vi "Controller Response Matrix Measurement Loop.vi"(7 "Sync Objects":T1, 8 "error in (no error)":errorcluster, 11 "FOFB Configuration":T5={"FOFB Parameters"={"Network"={"FOFB Controller IP"="", "LNLS Control Network IP"="", "LNLS Control Network Power Supplies TCP Port"=0, "LNLS Control Network FOFB Configuration TCP Port"=0, "Data Server TCP Port"=0, "Monitoring Data TCP Port"=0, "Configuration GUI TCP Port"=0, "TCP Listening Timeout"=0}, "Fast Acquisition"={"Acquisition Period"=0, "Data Buffer Size"=0}, "Response Matrix Measurement"={"Step Amplitude"=0.0, "Time Between Steps"=0, "Step Duration"=0, "Number of Averages"=0}, "Correction Algorithm"={"Correction Period"=0, "Reference Orbit Path"=path "", "Response Matrix Path"=path "", "Correction Matrix Path"=path "", "Horizontal Correction Factor"=0.0, "Vertical Correction Factor"=0.0, "Beam Current FOFB Threshold"=0.0, "Decouple H-V"=FALSE}, "Acquisition Network"=[], "Actuation Network"=[]}, "Number of Acquisition Chassis"=0, "Number of Actuation Chassis"=0, "Number of BPM Readings"=0, "BPM Reading Names"=[], "Selected BPM Readings"=[0, 1, 2, 3, 4, 5, 6, 7, 8, 9, 10, 11, 12, 13, 14, 15, 16, 17, 18, 19, 20, 21, 22, 23, 24, 25, 26, 27, 28, 29, 30, 31, 32, 33, 34, 35, 36, 37, 38, 39, 40, 41, 42, 43, 44, 45, 46, 47, 48, 49], "Number of Correctors"=0, "Corrector Names"=[], "Selected Correctors"=[0, 1, 2, 3, 4, 5, 6, 7, 8, 9, 10, 11, 12, 13, 14, 15, 16, 17, 18, 19, 20, 21, 22, 23, 24, 25, 26, 27, 28, 29, 30, 31, 32, 33, 34, 35, 36, 37, 38, 39, 40, 41, 42, 43, 44, 45, 46, 47, 48, 49], "Reference Orbit"=[], "Response Matrix"=[], "Correction Matrix"=[], "Acquisition Chassis Names"=[], "Actuation Chassis Names"=[], "Acquisition Variables"=[], "Actuation Variables"=[], "PS Matrix Mapping"=[], "Inverse PS Matrix Mapping"=[], "Response Matrix Beam Energy (MeV)"=0.0, "PID Parameters"=[], "BPM Planes"=[], "Corrector Planes"=[], "RMM Step Factor"=[]}) -> (0 "error out":errorcluster)   [LabVIEW 2011, in "Controller VIs.lvlib"]
uses:
  Controller VIs.lvlib
  Types Definitions/Type FOFB Configuration.ctl
  Types Definitions/Type FOFB Parameters.ctl
  Types Definitions/Type Network Configuration.ctl
  Types Definitions/Type FA Configuration.ctl
  Types Definitions/Type Response Matrix Measurement Configuration.ctl
  Types Definitions/Type Correction Algorithm Configuration.ctl
  Types Definitions/Type Acquisition Network Configuration.ctl
  Types Definitions/Type Actuation Network Configuration.ctl
  Types Definitions/Type PID Parameters.ctl
  Types Definitions/Type Synchronization Objects.ctl
  Types Definitions/Type Blocking Synchronization Objects.ctl
  Types Definitions/Type FA Request Parameters.ctl
  Types Definitions/Type BPM and PS select cluster.ctl
  Types Definitions/Type FA File Parameters.ctl
  Types Definitions/Type Monitoring Data.ctl
  Types Definitions/Type Diagnostics Data.ctl
  Types Definitions/Type CPU Loads Array.ctl
  Types Definitions/Type CPU Loads.ctl
  Types Definitions/Type Non-blocking Synchronization Objects.ctl
  Types Definitions/Type FOFB Variables.ctl
  Types Definitions/Type Actuation State.ctl
  <vilib>/Platform/TimedLoop/XDataNode/timing_clust.ctl
  <vilib>/Platform/TimedLoop/XDataNode/nitl_modes.ctl
  <vilib>/Platform/TimedLoop/XDataNode/wakeup.ctl
  Controller Global Variables/Monitoring Data.vi
  Controller Global Variables/LNLS Control FOFB Configuration Out.vi
  <vilib>/Platform/TimedLoop/XDataNode/XDataNode.xnode
  File VIs.lvlib
  Controller Global Variables.lvlib
  Type Definitions.lvlib
  <vilib>/Platform/TimedLoop/XDataNode/XDNodeRunTimeDep.lvlib
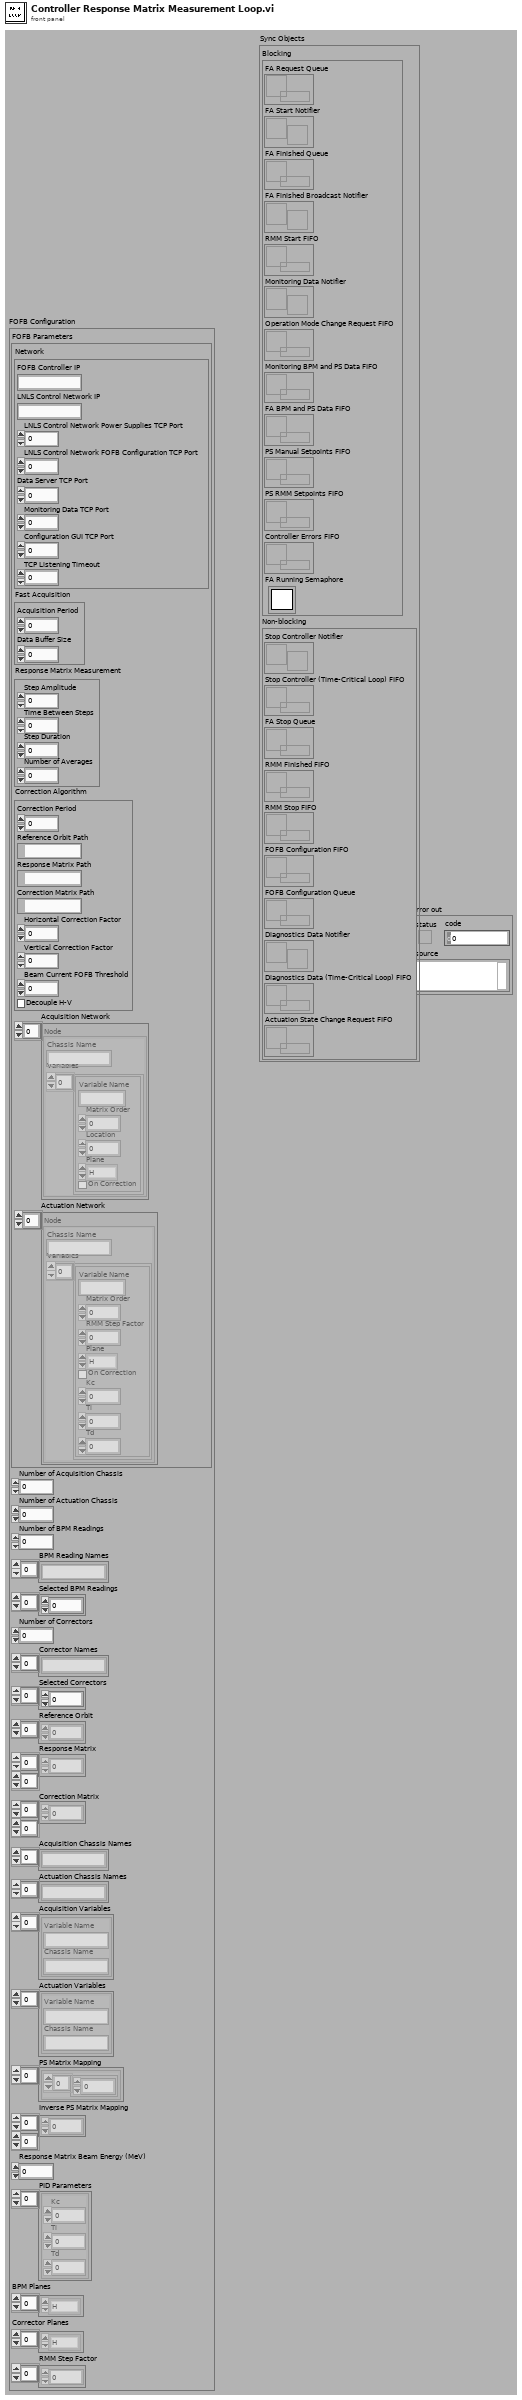
[diagram p1: front panel]
types:
  T1 = typedef "Type Definitions.lvlib/Type Synchronization Objects.ctl" = cluster{"Blocking":T2, "Non-blocking":T4}
  T2 = typedef "Type Definitions.lvlib/Type Blocking Synchronization Objects.ctl" = cluster{"FA Request Queue":refnum<queue>, "FA Start Notifier":refnum<notifier>, "FA Finished Queue":refnum<queue>, "FA Finished Broadcast Notifier":refnum<notifier>, "RMM Start FIFO":refnum<k33>, "Monitoring Data Notifier":refnum<notifier>, "Operation Mode Change Request FIFO":refnum<k33>, "Monitoring BPM and PS Data FIFO":refnum<k33>, "FA BPM and PS Data FIFO":refnum<k33>, "PS Manual Setpoints FIFO":refnum<k33>, "PS RMM Setpoints FIFO":refnum<k33>, "Controller Errors FIFO":refnum<k33>, "FA Running Semaphore":T3}
  T3 = typedef "Semaphore RefNum" = refnum<k1>
  T4 = typedef "Type Definitions.lvlib/Type Non-blocking Synchronization Objects.ctl" = cluster{"Stop Controller Notifier":refnum<notifier>, "Stop Controller (Time-Critical Loop) FIFO":refnum<k33>, "FA Stop Queue":refnum<queue>, "RMM Finished FIFO":refnum<k33>, "RMM Stop FIFO":refnum<k33>, "FOFB Configuration FIFO":refnum<k33>, "FOFB Configuration Queue":refnum<queue>, "Diagnostics Data Notifier":refnum<notifier>, "Diagnostics Data (Time-Critical Loop) FIFO":refnum<k33>, "Actuation State Change Request FIFO":refnum<k33>}
  T5 = typedef "Type Definitions.lvlib/Type FOFB Configuration.ctl" = cluster{"FOFB Parameters":T6, "Number of Acquisition Chassis":i32, "Number of Actuation Chassis":i32, "Number of BPM Readings":i32, "BPM Reading Names":string[], "Selected BPM Readings":u32[], "Number of Correctors":i32, "Corrector Names":string[], "Selected Correctors":u32[], "Reference Orbit":dbl[], "Response Matrix":dbl[][], "Correction Matrix":dbl[][], "Acquisition Chassis Names":string[], "Actuation Chassis Names":string[], "Acquisition Variables":cluster{"Variable Name":string, "Chassis Name":string}[], "Actuation Variables":cluster{"Variable Name":string, "Chassis Name":string}[], "PS Matrix Mapping":cluster{u32[]}[], "Inverse PS Matrix Mapping":u32[][], "Response Matrix Beam Energy (MeV)":dbl, "PID Parameters":T13[], "BPM Planes":enum8{"H", "V"}[], "Corrector Planes":enum8{"H", "V"}[], "RMM Step Factor":dbl[]}
  T6 = typedef "Type Definitions.lvlib/Type FOFB Parameters.ctl" = cluster{"Network":T7, "Fast Acquisition":T8, "Response Matrix Measurement":T9, "Correction Algorithm":T10, "Acquisition Network":T11, "Actuation Network":T12}
  T7 = typedef "Type Definitions.lvlib/Type Network Configuration.ctl" = cluster{"FOFB Controller IP":string, "LNLS Control Network IP":string, "LNLS Control Network Power Supplies TCP Port":u16, "LNLS Control Network FOFB Configuration TCP Port":u16, "Data Server TCP Port":u16, "Monitoring Data TCP Port":u16, "Configuration GUI TCP Port":u16, "TCP Listening Timeout":i32}
  T8 = typedef "Type Definitions.lvlib/Type FA Configuration.ctl" = cluster{"Acquisition Period":u32, "Data Buffer Size":u32}
  T9 = typedef "Type Definitions.lvlib/Type Response Matrix Measurement Configuration.ctl" = cluster{"Step Amplitude":dbl, "Time Between Steps":u32, "Step Duration":u32, "Number of Averages":u32}
  T10 = typedef "Type Definitions.lvlib/Type Correction Algorithm Configuration.ctl" = cluster{"Correction Period":u32, "Reference Orbit Path":path, "Response Matrix Path":path, "Correction Matrix Path":path, "Horizontal Correction Factor":dbl, "Vertical Correction Factor":dbl, "Beam Current FOFB Threshold":dbl, "Decouple H-V":bool}
  T11 = typedef "Type Definitions.lvlib/Type Acquisition Network Configuration.ctl" = cluster{"Chassis Name":string, "Variables":cluster{"Variable Name":string, "Matrix Order":u32, "Location":dbl, "Plane":enum8{"H", "V"}, "On Correction":bool}[]}[]
  T12 = typedef "Type Definitions.lvlib/Type Actuation Network Configuration.ctl" = cluster{"Chassis Name":string, "Variables":cluster{"Variable Name":string, "Matrix Order":u32, "RMM Step Factor":dbl, "Plane":enum8{"H", "V"}, "On Correction":bool, "Kc":dbl, "Ti":dbl, "Td":dbl}[]}[]
  T13 = typedef "Type Definitions.lvlib/Type PID Parameters.ctl" = cluster{"Kc":fxp<+/-,16,8>, "Ti":fxp<+/-,16,8>, "Td":fxp<+/-,16,8>}
  T14 = typedef "XDNodeRunTimeDep.lvlib/timing_clust.ctl" = cluster{"Expected End [f-1]":u64, "Actual End [f-1]":u64, "Finished Late? [f-1]":bool, "Expected End [i-1]":u64, "Actual End [i-1]":u64, "Finished Late? [i-1]":bool, "Expected Start [i]":u64, "Actual Start [i]":u64, "Expected Start [f]":u64, "Actual Start [f]":u64, "Source Name":string, "Structure Name":string, "Period":i64, "Deadline":i64, "Offset":i64, "Start":i64, "Priority":i32, "Timeout":i32, "Mode":T15, "Wakeup Reason":T16, "Error":errorcluster, "Source Type":string, "Secondary Source Type":string, "Global End Time":u64, "Global Start Time":u64, "Frame Duration":u64, "Iteration Duration":u64, "Assigned CPU":i32, "I/O Scan Engine Mode":u32}
  T15 = typedef "XDNodeRunTimeDep.lvlib/nitl_modes.ctl" = enum32{"No Change", "Process missed periods, maintain original phase", "Discard missed periods, maintain original phase", "Process missed periods, ignore original phase", "Discard missed periods, ignore original phase"}
  T16 = typedef "XDNodeRunTimeDep.lvlib/wakeup.ctl" = enum32{"Normal", "Aborted", "Asynchronous wakeup", "Timing source error", "Timed loop error", "Timeout"}
  T17 = typedef "Type Definitions.lvlib/Type BPM and PS select cluster.ctl" = cluster{"BPM index array":u32[], "PS index array ":u32[]}
  T18 = typedef "Type Definitions.lvlib/Type FA Request Parameters.ctl" = cluster{"Number of Samples":u32, "BPM and PS Selection":T17, "Filename":string}
  T19 = typedef "Type Definitions.lvlib/Type Monitoring Data.ctl" = cluster{"Timestamp":timestamp, "BPM Readings":dbl[], "PS Readings":dbl[], "PS FOFB Setpoints":dbl[], "PS Status per Rack":u8[], "PS ON-OFF per Rack":u8[], "Operation Mode":enum16{"Idle Mode", "Error Mode", "Manual Mode", "FOFB Mode", "RMM Mode"}, "Diagnostics Data":T20, "Controller Status Table":i32[]}
  T20 = typedef "Type Definitions.lvlib/Type Diagnostics Data.ctl" = cluster{"Time-Critical Loop Missed Iterations":u32, "Time-Critical Loop Execution Time (usec)":u32, "FA Buffer Usage":u32, "Available Memory (bytes)":u32, "CPU Loads Array":T21}
  T21 = typedef "Type Definitions.lvlib/Type CPU Loads Array.ctl" = T22[]
  T22 = typedef "Type Definitions.lvlib/Type CPU Loads.ctl" = cluster{"Total (%)":dbl, "Time Critical (%)":dbl, "Timed Structures (%)":dbl, "High (%)":dbl, "Above Normal (%)":dbl, "Normal (%)":dbl, "Background (%)":dbl, "Idle (%)":dbl, "ISR (%)":dbl}
  T23 = cluster{"Operation Mode":enum16{"Idle Mode", "Error Mode", "Manual Mode", "FOFB Mode", "RMM Mode"}, "Correction Period (usec)":i32, "Beam Energy (MeV)":sgl, "Beam Current (mA)":sgl}
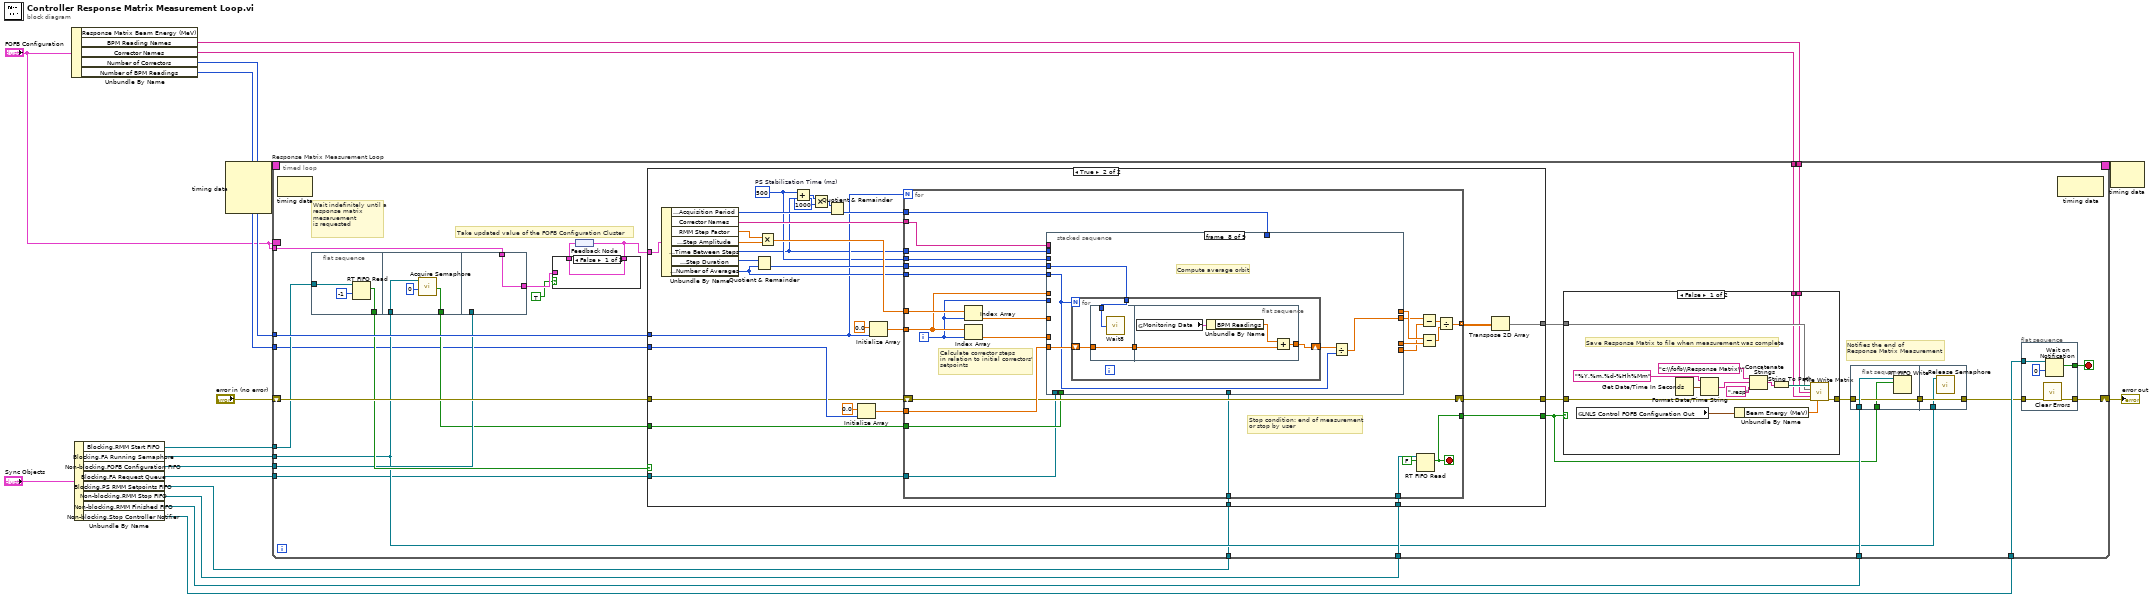
[diagram p0: block diagram]
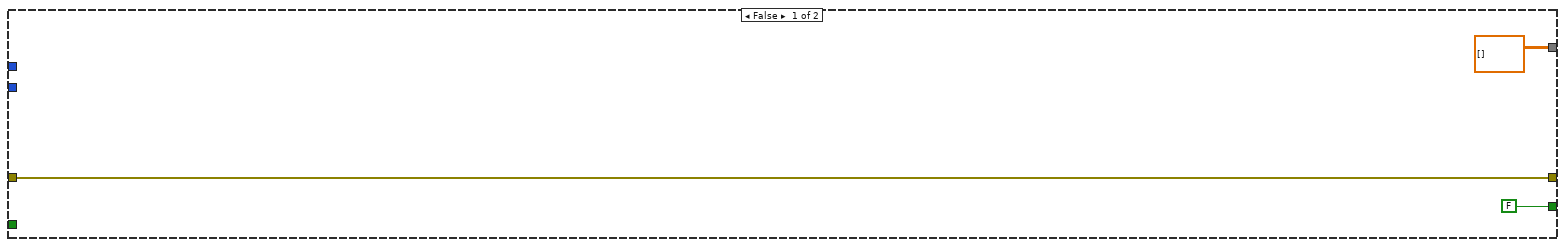
[diagram p3: hidden frame]
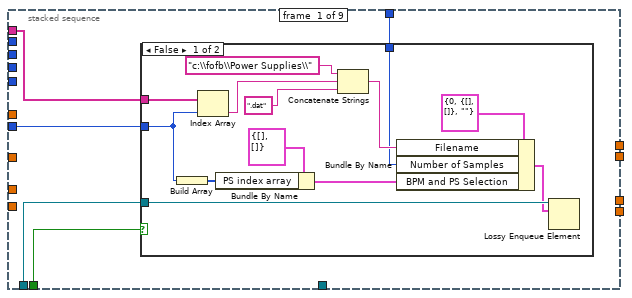
[diagram p4: hidden frame]
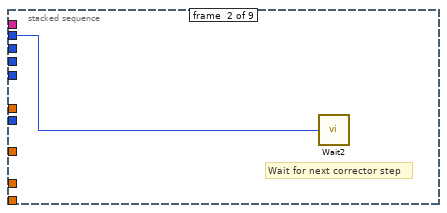
[diagram p6: hidden frame]
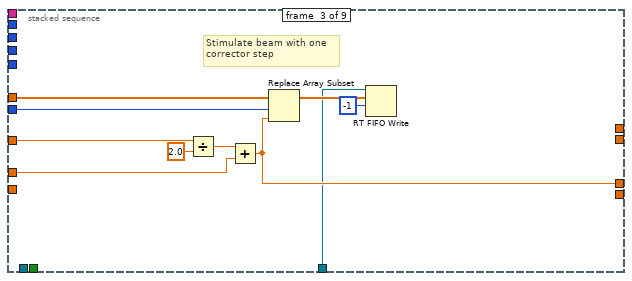
[diagram p7: hidden frame]
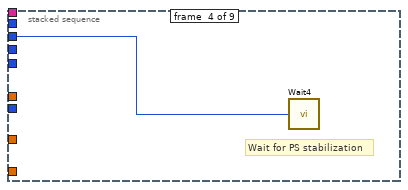
[diagram p8: hidden frame]
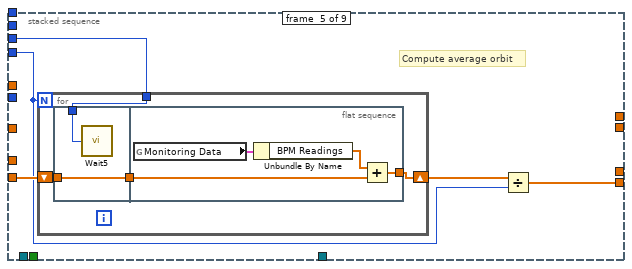
[diagram p9: hidden frame]
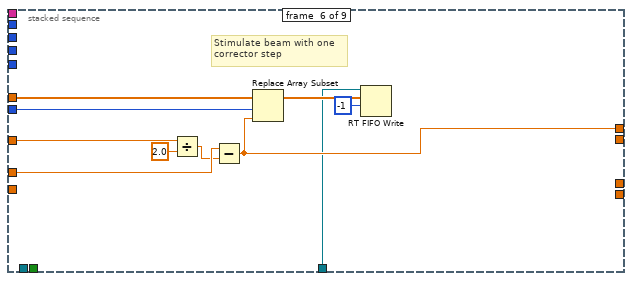
[diagram p10: hidden frame]
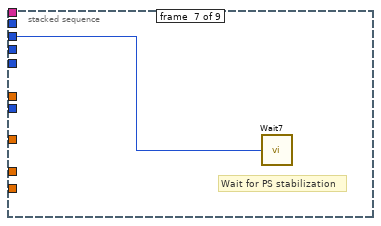
[diagram p11: hidden frame]
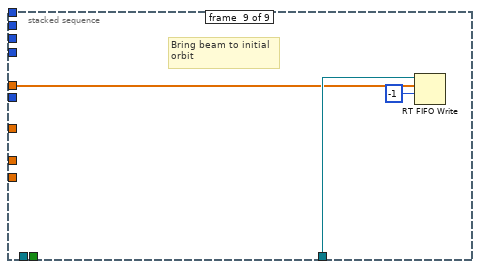
[diagram p12: hidden frame]
diagram:
  n1 = Unbundle By Name("FOFB Configuration") -> ("BPM Reading Names"=w10:string[], "Corrector Names"=w9:string[], "Number of Correctors"=w12:i32, "Number of BPM Readings"=w11:i32)  [unwired: 1 out]
  n2 = Unbundle By Name("Sync Objects") -> ("Blocking.RMM Start FIFO"=w7:refnum<k33>, "Blocking.FA Running Semaphore"=w6:T3, "Non-blocking.FOFB Configuration FIFO"=w8:refnum<k33>, "Blocking.FA Request Queue"=w5:refnum<queue>, "Blocking.PS RMM Setpoints FIFO"=w3:refnum<k33>, "Non-blocking.RMM Stop FIFO"=w13:refnum<k33>, "Non-blocking.RMM Finished FIFO"=w15:refnum<k33>, "Non-blocking.Stop Controller Notifier"=w14:refnum<notifier>)
  n3 = node-c288() -> (w2:T14)  [unwired: 4 in]
  n4 = timed-loop "Response Matrix Measurement Loop" {
    shift-right: [w31] -> w18
    shift-left: "error in (no error)" -> [w36]
    tunnel: w12 -> [w46]
    tunnel: w11 -> [w19]
    tunnel: w10 -> [w45]
    tunnel: w9 -> [w44]
    tunnel: w15 -> [w39]
    tunnel: w14 -> [w43]
    tunnel: w13 -> [w40]
    tunnel: w8 -> [w34]
    tunnel: w7 -> [w33]
    border: "FOFB Configuration" -> [_]
    tunnel: w6 -> [w25]
    tunnel: w5 -> [w24]
    tunnel: "FOFB Configuration" -> [w22]
    tunnel: w3 -> [w20]
    timing: w2 -> [_]
    timing-out: [_] -> w1
    stop <- w32 stop-if-true
    # "Take updated value of the FOFB Configuration Cluster"
    # "Notifies the end of\nResponse Matrix Measurement"
    # "Wait indefinitely until a response matrix mesaruement\nis requested"
    n5 = node-c288() -> ()  [unwired: 1 in, 1 out]
    n6 = flat-sequence {
      tunnel: w33 -> [w57]
      tunnel: [w56] -> w35
      tunnel: w25 -> [w61]
      tunnel: [w59] -> w27
      tunnel: w34 -> [_]
      tunnel: [w62] -> w23
      tunnel: w22 -> [w62]
      frame #0 {
        n7 = RT FIFO Read(0:w57, 2:-1 ("timeout in ms (-1)")) -> (9:w56:bool)  [unwired: 2 in, 4 out]
      }
      frame #1 {
        n8 = call <vilib>:"Acquire Semaphore.vi"("ms timeout (-1)"=0, "semaphore"=w61) -> ("timed out"=w59:bool)  [unwired: 3 in, 2 out]
      }
      frame #2 {
      }
    }
    n9 = feedback #1() -> (w30:T5)
    n10 = case shown="False" TRUE {
      tunnel: w23 -> [_ w50]
      tunnel: w30 -> [w49 _]
      tunnel: [w49 w50] -> w29
      frame False {
      }
      frame True {
      }
    }
    n11 = feedback-in #1(w29) -> ()
    n12 = case shown="True" w35 {
      tunnel: w36 -> [w70 w88]
      tunnel: [w70 w94] -> w42
      tunnel: [FALSE ("Calculation Stopped?") w93] -> w37
      tunnel: [dbl[][] [] ("Response Matrix") w91] -> w41
      tunnel: w46 -> [_ w76]
      tunnel: w19 -> [_ w90]
      tunnel: w40 -> [_ w85]
      tunnel: w29 -> [_ w84]
      tunnel: w27 -> [_ w82]
      tunnel: w24 -> [_ w81]
      tunnel: w20 -> [_ w79]
      frame False {
      }
      frame True {
        w73 = u32 500  # PS Stabilization Time (ms)
        n13 = Unbundle By Name(w84) -> ("FOFB Parameters.Fast Acquisition.Acquisition Period"=w78:u32, "Corrector Names"=w80:string[], "RMM Step Factor"=w83:dbl[], "FOFB Parameters.Response Matrix Measurement.Step Amplitude"=w99:dbl, "FOFB Parameters.Response Matrix Measurement.Time Between Steps"=w72:u32, "FOFB Parameters.Response Matrix Measurement.Step Duration"=w87:u32, "FOFB Parameters.Response Matrix Measurement.Number of Averages"=w86:u32)
        n14 = Quotient & Remainder(x=w87, y=w86) -> (floor(x/y)=w95:u32)  [unwired: 1 out]
        n15 = Multiply(x=w83, y=w99) -> (x*y=w98:dbl[])
        n16 = Add(x=w73, y=w72) -> (x+y=w74:u32)
        n17 = Multiply(x=w74, y=u32 1000) -> (x*y=w75:u32)
        n18 = Quotient & Remainder(x=w75, y=w78) -> (floor(x/y)=w77:u32)  [unwired: 1 out]
        n19 = Initialize Array(0.0 ("element"), w90) -> (w96:dbl[])
        n20 = Initialize Array(0.0 ("element"), w76) -> (w89:dbl[])
        n21 = for {
          N: w76 -> [_]
          tunnel: w89 -> [w125]
          tunnel: w98 -> [w126]
          shift-right: [w111] -> w94
          shift-left: w88 -> [w111]
          tunnel: w86 -> [w124]
          tunnel: w96 -> [w123]
          tunnel: w95 -> [w122]
          tunnel: [w110] -> w92 mode=indexing
          tunnel: w72 -> [w113]
          tunnel: [w101] -> w93
          tunnel: w73 -> [w112]
          tunnel: w85 -> [w109]
          tunnel: w82 -> [w107]
          tunnel: w81 -> [w106]
          tunnel: w80 -> [w105]
          tunnel: w79 -> [w103]
          tunnel: w77 -> [w102]
          i -> [w108]
          stop <- w101 stop-if-true
          # "Stop condition: end of measurement\nor stop by user"
          # "Calculate corrector steps\nin relation to initial correctors'\nsetpoints"
          n22 = Index Array(array=w126, index=w108) -> (element=w115:dbl)
          n23 = Index Array(array=w125, index=w108) -> (element=w114:dbl)
          n24 = stacked-sequence {
            tunnel: w125 -> [_ _ w151 _ _ w181 _ _ w198]
            tunnel: [_ _ _ _ _ w175 _ _ _] -> w118
            tunnel: [_ _ _ _ _ _ _ w183 _] -> w116
            tunnel: w124 -> [_ _ _ _ w157 _ _ w184 _]
            tunnel: [_ _ _ _ w160 _ _ _ _] -> w117
            tunnel: [_ _ w149 _ _ _ _ _ _] -> w119
            tunnel: w123 -> [_ _ _ _ w159 _ _ w186 _]
            tunnel: w122 -> [_ _ _ _ w158 _ _ w185 _]
            tunnel: w115 -> [_ _ w155 _ _ w177 _ _ _]
            tunnel: w114 -> [_ _ w152 _ _ w179 _ _ _]
            tunnel: w108 -> [w128 _ w150 _ _ w180 _ _ _]
            tunnel: w113 -> [_ w145 _ _ _ _ _ _ _]
            tunnel: w112 -> [_ _ _ w156 _ _ w182 _ _]
            tunnel: w107 -> [w130 _ _ _ _ _ _ _ _]
            tunnel: w106 -> [w129 _ _ _ _ _ _ _ _]
            tunnel: w105 -> [w131 _ _ _ _ _ _ _ _]
            tunnel: w103 -> [_ _ w146 _ _ w172 _ _ w199]
            tunnel: w102 -> [w127 _ _ _ _ _ _ _ _]
            frame #0 {
              n25 = case shown="False" w130 {
                tunnel: w129 -> [w144 _]
                tunnel: w128 -> [w135 _]
                tunnel: w131 -> [w136 _]
                tunnel: w127 -> [w132 _]
                frame False {
                  n26 = Build Array(w135) -> (w139:i32[])
                  n27 = Index Array(array=w136, index=w135) -> (element=w134:string)
                  n28 = Bundle By Name(cluster=T17 {"BPM index array"=[], "PS index array "=[]} ("BPM and PS Selection"), "PS index array"=w139) -> (w140:T17)
                  n29 = Concatenate Strings("c:\\fofb\\Power Supplies\\" ("string"), w134, ".dat" ("Variable Name")) -> (w133:string)
                  n30 = Bundle By Name(cluster=T18 {"Number of Samples"=0, "BPM and PS Selection"={"BPM index array"=[], "PS index array "=[]}, "Filename"=""} ("notification"), "Filename"=w133, "Number of Samples"=w132, "BPM and PS Selection"=w140) -> (w142:T18)
                  n31 = Lossy Enqueue Element(queue=w144, element=w142) -> ()  [unwired: 1 in, 4 out]
                }
                frame True {
                }
              }
            }
            frame #1 {
              # "Wait for next corrector step"
              n32 = call "Wait2"("Count(mSec)"=w145) -> ()  [unwired: 1 out]
            }
            frame #2 {
              # "Stimulate beam with one\ncorrector step"
              n33 = Divide(x=w155, y=2.0) -> (x/y=w153:dbl)
              n34 = Add(x=w153, y=w152) -> (x+y=w149:dbl)
              n35 = Replace Array Subset(array=w151, new element=w149, index=w150) -> (w147:dbl[])
              n36 = RT FIFO Write(0:w146, 1:w147, 2:-1 ("timeout in ms (0)")) -> ()  [unwired: 2 in, 4 out]
            }
            frame #3 {
              # "Wait for PS stabilization"
              n37 = call "Wait4"("Count(mSec)"=w156) -> ()  [unwired: 1 out]
            }
            frame #4 {
              # "Compute average orbit"
              n38 = for {
                N: w157 -> [_]
                shift-right: [w163] -> w161
                shift-left: w159 -> [w165]
                tunnel: w158 -> [w162]
                n39 = flat-sequence {
                  tunnel: w165 -> [w167]
                  tunnel: [w167] -> w164
                  tunnel: w162 -> [w166]
                  tunnel: w164 -> [w170]
                  tunnel: [w171] -> w163
                  frame #0 {
                    n40 = call "Wait5"("Count(mSec)"=w166) -> ()  [unwired: 1 out]
                  }
                  frame #1 {
                    n41 = global read "Monitoring Data.vi" "Monitoring Data"() -> (w169:T19)
                    n42 = Unbundle By Name(w169) -> ("BPM Readings"=w168:dbl[])
                    n43 = Add(x=w168, y=w170) -> (x+y=w171:dbl[])
                  }
                }
              }
              n44 = Divide(x=w161, y=w157) -> (x/y=w160:dbl[])
            }
            frame #5 {
              # "Stimulate beam with one\ncorrector step"
              n45 = Divide(x=w177, y=2.0) -> (x/y=w176:dbl)
              n46 = Subtract(x=w179, y=w176) -> (x-y=w175:dbl)
              n47 = Replace Array Subset(array=w181, new element=w175, index=w180) -> (w174:dbl[])
              n48 = RT FIFO Write(0:w172, 1:w174, 2:-1 ("timeout in ms (0)")) -> ()  [unwired: 2 in, 4 out]
            }
            frame #6 {
              # "Wait for PS stabilization"
              n49 = call "Wait7"("Count(mSec)"=w182) -> ()  [unwired: 1 out]
            }
            frame #7 {
              # "Compute average orbit"
              n50 = for {
                N: w184 -> [_]
                shift-right: [w189] -> w187
                shift-left: w186 -> [w191]
                tunnel: w185 -> [w188]
                n51 = flat-sequence {
                  tunnel: w191 -> [w193]
                  tunnel: [w193] -> w190
                  tunnel: w188 -> [w192]
                  tunnel: w190 -> [w196]
                  tunnel: [w197] -> w189
                  frame #0 {
                    n52 = call "Wait8"("Count(mSec)"=w192) -> ()  [unwired: 1 out]
                  }
                  frame #1 {
                    n53 = global read "Monitoring Data.vi" "Monitoring Data"() -> (w195:T19)
                    n54 = Unbundle By Name(w195) -> ("BPM Readings"=w194:dbl[])
                    n55 = Add(x=w194, y=w196) -> (x+y=w197:dbl[])
                  }
                }
              }
              n56 = Divide(x=w187, y=w184) -> (x/y=w183:dbl[])
            }
            frame #8 {
              # "Bring beam to initial\norbit"
              n57 = RT FIFO Write(0:w199, 1:w198, 2:-1 ("timeout in ms (0)")) -> ()  [unwired: 2 in, 4 out]
            }
          }
          n58 = RT FIFO Read(0:w109, 1:FALSE ("element")) -> (9:w101:bool)  [unwired: 2 in, 4 out]
          n59 = Subtract(x=w116, y=w117) -> (x-y=w120:dbl[])
          n60 = Subtract(x=w118, y=w119) -> (x-y=w121:dbl)
          n61 = Divide(x=w120, y=w121) -> (x/y=w110:dbl[])
        }
        n62 = Transpose 2D Array(2D array=w92) -> (transposed array=w91:dbl[][])
      }
    }
    n63 = case shown="False" w37 {
      tunnel: w42 -> [w214 w215]
      tunnel: w41 -> [w208 _]
      tunnel: w45 -> [w205 _]
      tunnel: w44 -> [w204 _]
      tunnel: [w202 w215] -> w38
      frame False {
        # "Save Response Matrix to file when measurement was complete"
        n64 = global read "LNLS Control FOFB Configuration Out.vi" "LNLS Control FOFB Configuration Out"() -> (w201:T23)
        n65 = Get Date/Time In Seconds() -> (seconds since 1Jan1904=w212:timestamp)
        n66 = Format Date/Time String(time format string (%c)="%Y.%m.%d-%Hh%Mm", seconds (now)=w212) -> (date/time string=w213:string)  [unwired: 1 in]
        n67 = Unbundle By Name(w201) -> ("Beam Energy (MeV)"=w203:sgl)
        n68 = Concatenate Strings("c:\\fofb\\Response Matrix\\", w213, ".resp" ("string")) -> (w210:string)
        n69 = String To Path(string=w210) -> (path=w209:path)
        n70 = call "File Write Matrix.vi"("file path (dialog if empty)"=w209, "Matrix"=w208, "Row Names"=w205, "Column Names"=w204, "error in (no error)"=w214, "Beam Energy (MeV)"=w203) -> ("error out"=w202:errorcluster)  [unwired: 9 in]
      }
      frame True {
        # "If the Response Matrix Measurement was aborted, all data is ignored."
      }
    }
    n71 = flat-sequence {
      tunnel: w39 -> [w65]
      tunnel: w38 -> [w64]
      tunnel: w37 -> [w63]
      tunnel: [w64] -> w26
      tunnel: [w67] -> w28
      tunnel: w26 -> [w67]
      tunnel: w25 -> [w66]
      frame #0 {
        n72 = RT FIFO Write(0:w65, 1:w63) -> ()  [unwired: 3 in, 4 out]
      }
      frame #1 {
        n73 = call <vilib>:"Release Semaphore.vi"("semaphore"=w66) -> ()  [unwired: 5 in, 2 out]
      }
    }
    n74 = flat-sequence {
      tunnel: w43 -> [w54]
      tunnel: w28 -> [w52]
      tunnel: [w53] -> w32
      tunnel: [w51] -> w31
      frame #0 {
        n75 = call <vilib>:"Clear Errors.vi"("error in (no error)"=w52) -> ("error out"=w51:errorcluster)  [unwired: 6 in]
        n76 = Wait on Notification(notifier=w54, timeout in ms (-1)=0) -> (notification=w53:bool)  [unwired: 2 in, 3 out]
      }
    }
    n77 = node-c288() -> ()  [unwired: 1 in, 1 out]
  }
  "error out" <- w18
  n78 = node-c288(w1) -> ()  [unwired: 1 out]
